vi "Trainging_Program_redesign_TV_White.vi"() -> ()   [LabVIEW 2014]
uses:
  <vilib>/Utility/file.llb/Write To Spreadsheet File (I64).vi
  <vilib>/Utility/file.llb/Write To Spreadsheet File (DBL).vi
  NeuroSky_Dll_Call/Debug/NeuroSky_Dll_Call.dll
panel:
  out "큐사인":bool
  out "실험종료":bool=TRUE
  out "icon_전원":bool
  out "icon_음향업":bool
  out "icon_체널업":bool
  out "icon_음향다운":bool
  out "icon_체널다운":bool=TRUE
  out "icon_전체종료":bool
  out "error out":errorcluster={"status"=TRUE, "code"=10, "source"="Create Folder in Trainging_Set_For_ LDA_Matrix_RSVP.vi<APPEND>\nC:\\Emotion_Research\\_Training_Test(LDA)\\2014-08-30"}
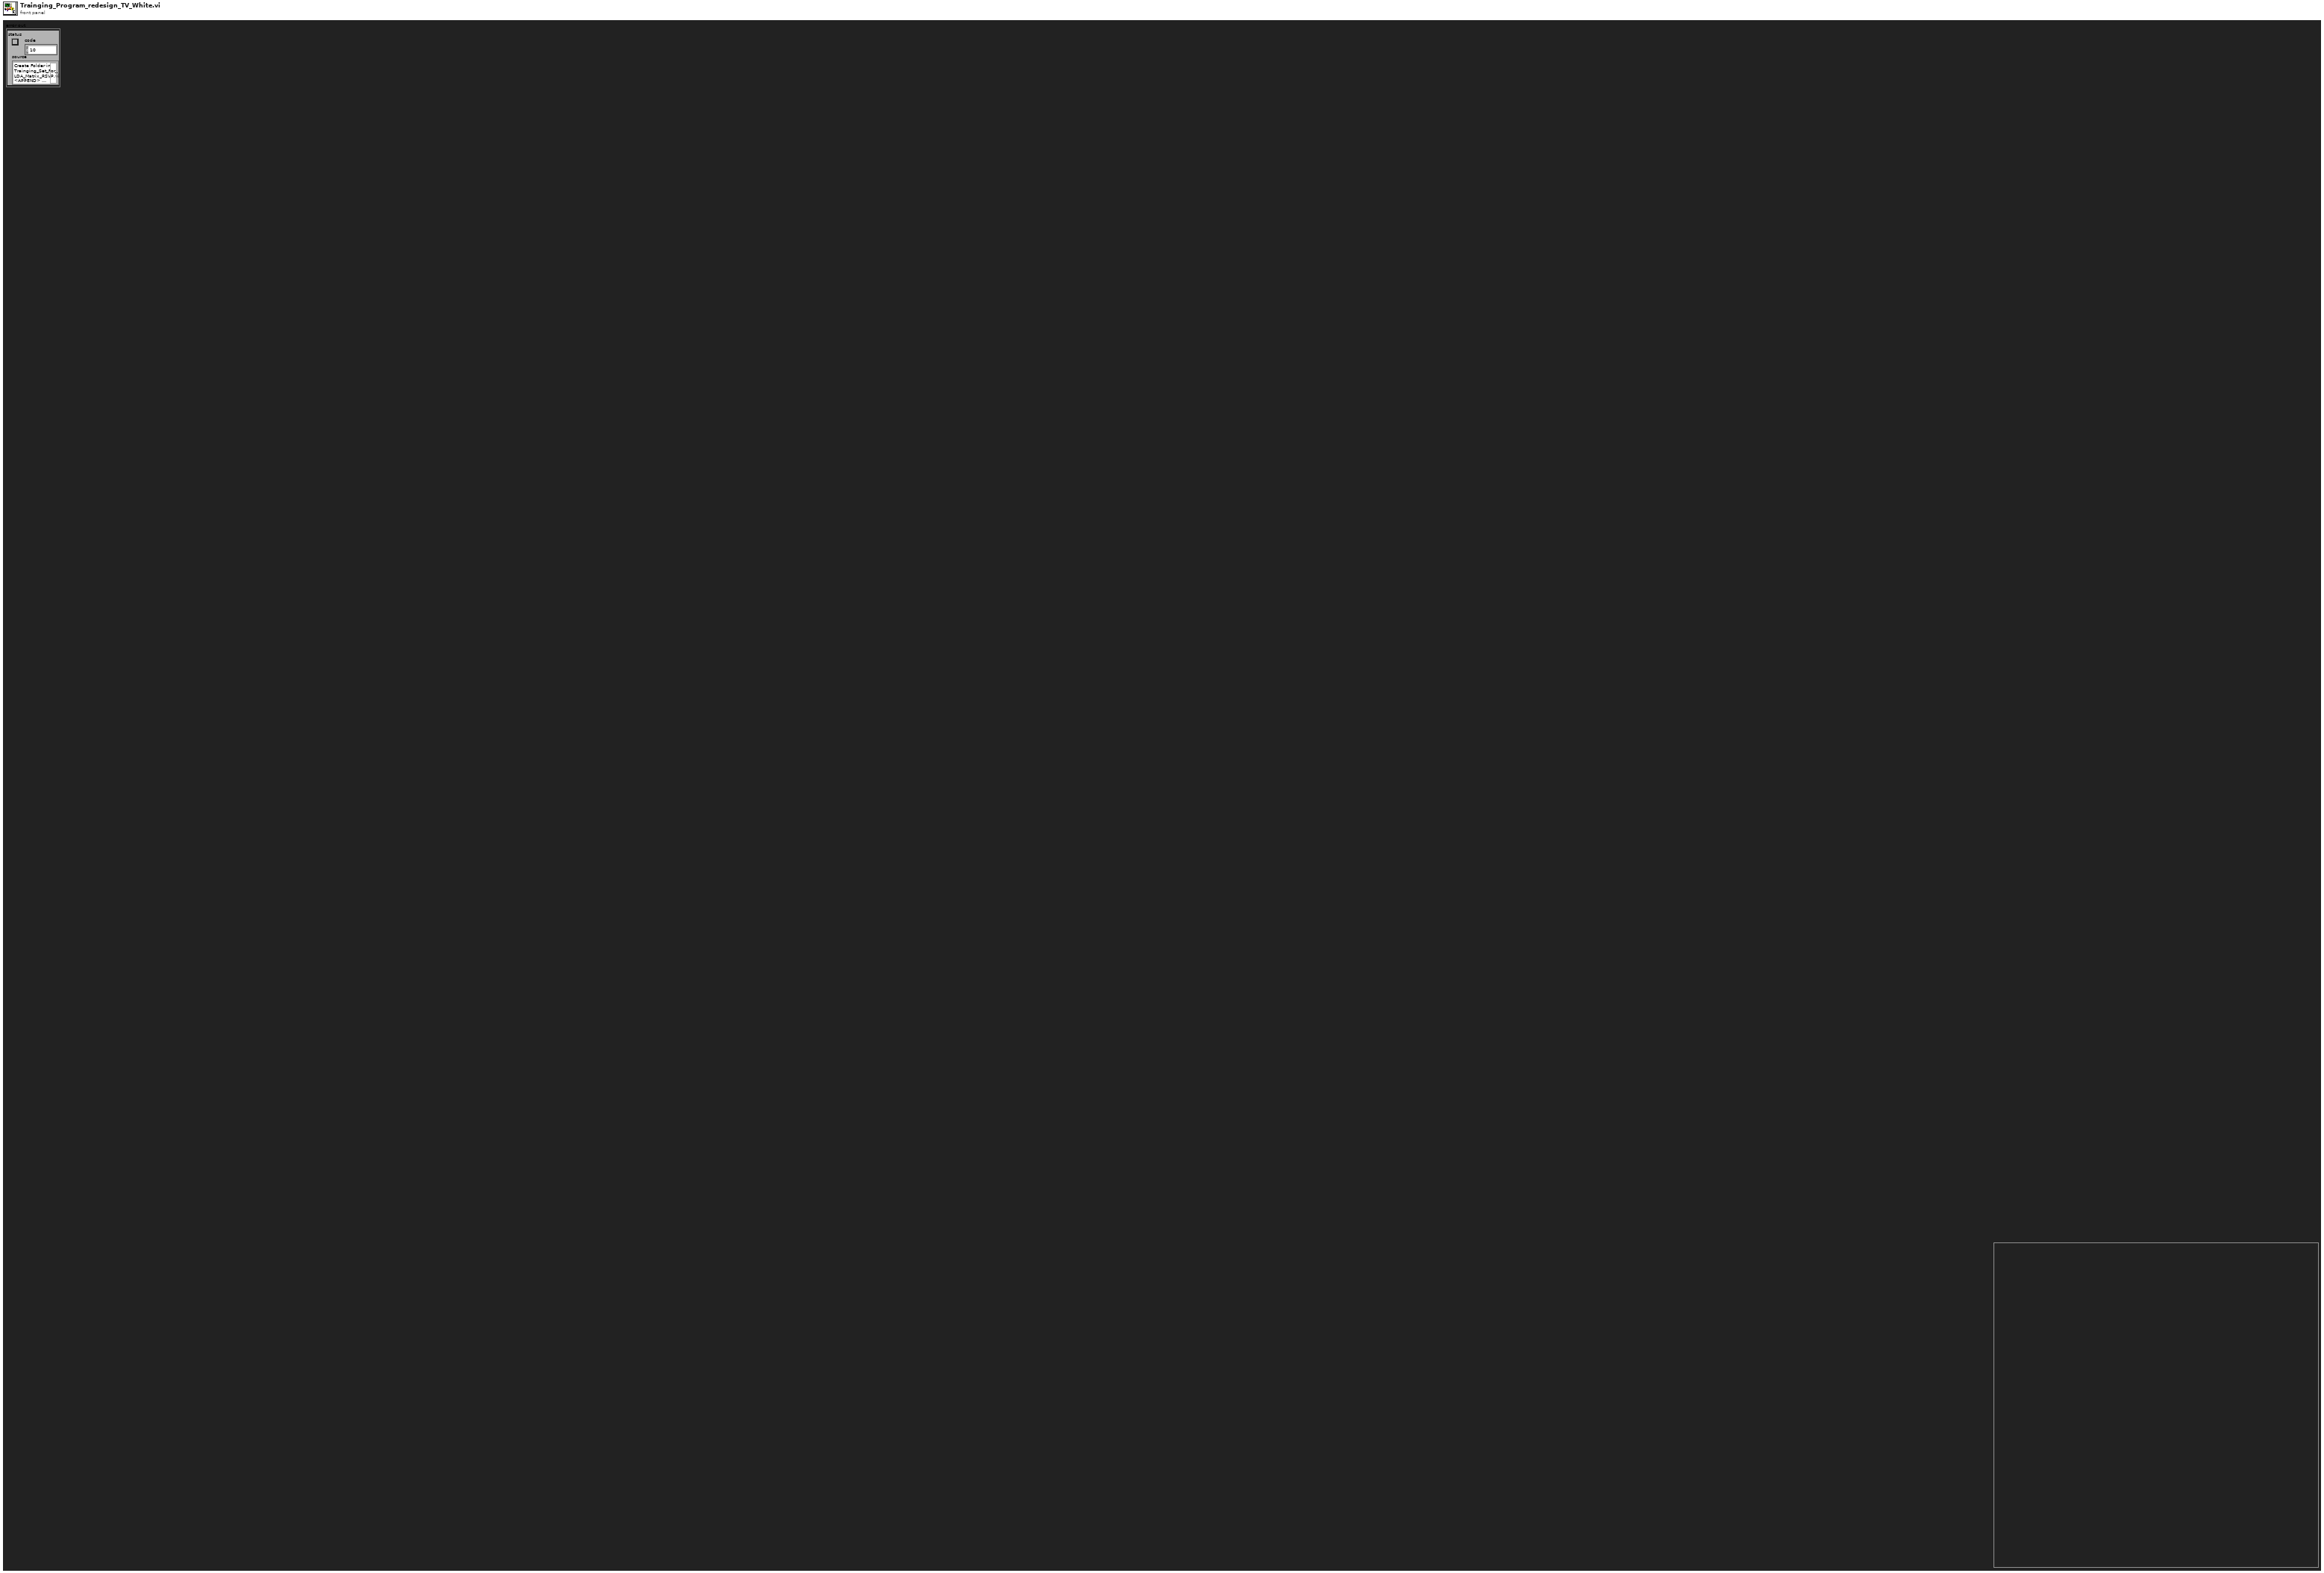
[diagram p1: front panel]
types:
  T1 = typedef "NI_Matrix.lvlib/RealMatrix.ctl" = dbl[][]
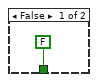
[diagram p2: hidden frame]
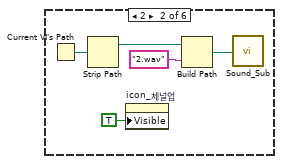
[diagram p3: hidden frame]
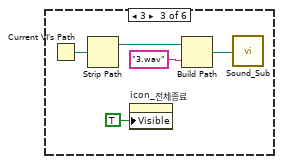
[diagram p4: hidden frame]
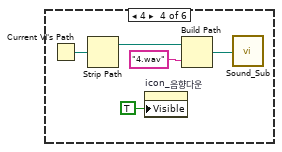
[diagram p5: hidden frame]
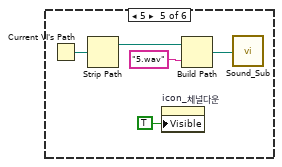
[diagram p6: hidden frame]
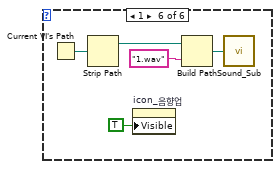
[diagram p7: hidden frame]
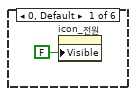
[diagram p8: hidden frame]
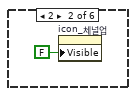
[diagram p9: hidden frame]
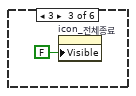
[diagram p10: hidden frame]
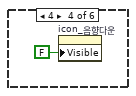
[diagram p11: hidden frame]
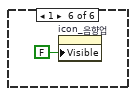
[diagram p12: hidden frame]
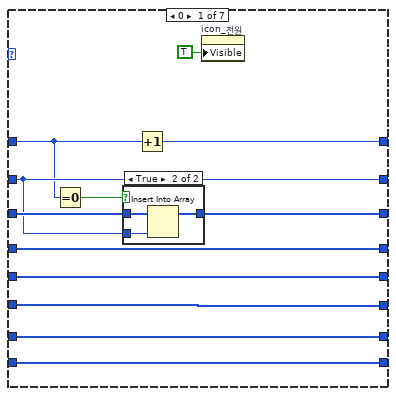
[diagram p14: hidden frame]
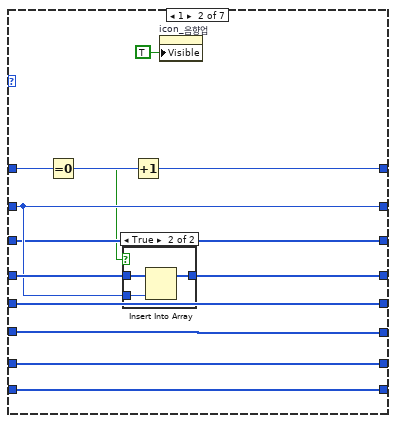
[diagram p16: hidden frame]
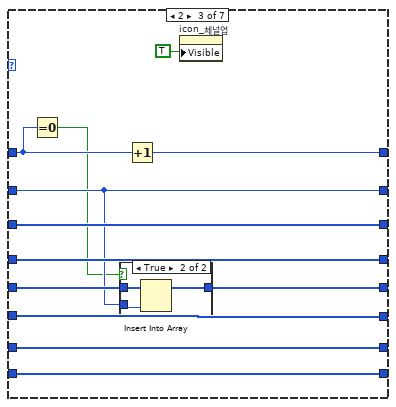
[diagram p18: hidden frame]
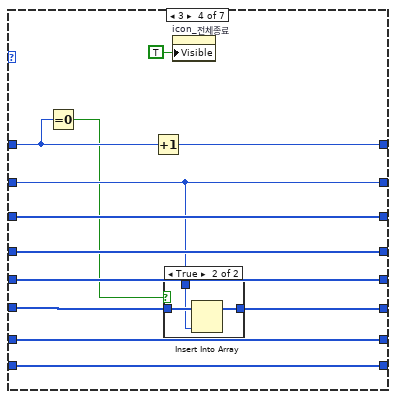
[diagram p20: hidden frame]
diagram:
  w8 = 500 ("Position:Left")
  w1 = FALSE ("Visible")
  # "0 = 온도/전원\n1 = 자판/음향업\n2 = 침대/체널업\n3 = 용변/전체종료\n4 = 기계/음향다운\n5 = 응급/체널다운"
  n1 = property on="icon_음향다운" class="Bool (strict)"("Left"=w8, "Top"=w8) -> ()  [unwired: 2 in, 2 out]
  n2 = property on="icon_음향업" class="Bool (strict)"("Left"=w8, "Top"=w8) -> ()  [unwired: 2 in, 2 out]
  n3 = property on="icon_체널업" class="Bool (strict)"("Left"=w8, "Top"=w8) -> ()  [unwired: 2 in, 2 out]
  n4 = property on="icon_체널다운" class="Bool (strict)"("Left"=w8, "Top"=w8) -> ()  [unwired: 2 in, 2 out]
  n5 = property on="icon_전원" class="Bool (strict)"("Left"=w8, "Top"=w8) -> ()  [unwired: 2 in, 2 out]
  n6 = property on="icon_전체종료" class="Bool (strict)"("Left"=w8, "Top"=w8) -> ()  [unwired: 2 in, 2 out]
  n7 = property on="실험종료" class="Bool (strict)"("Left"=200 ("Position:Left"), "Top"=600 ("Position:Top")) -> ()  [unwired: 2 in, 2 out]
  n8 = property on="큐사인" class="Bool (strict)"("Left"=w8, "Top"=w8) -> ()  [unwired: 2 in, 2 out]
  n9 = property on="큐사인" class="Bool (strict)"("Visible"=w1) -> ()  [unwired: 2 in, 2 out]
  n10 = property on="실험종료" class="Bool (strict)"("Visible"=w1) -> ()  [unwired: 2 in, 2 out]
  n11 = property on="icon_음향다운" class="Bool (strict)"("Visible"=w1) -> ()  [unwired: 2 in, 2 out]
  n12 = property on="icon_전원" class="Bool (strict)"("Visible"=w1) -> ()  [unwired: 2 in, 2 out]
  n13 = property on="icon_음향업" class="Bool (strict)"("Visible"=w1) -> ()  [unwired: 2 in, 2 out]
  n14 = property on="icon_체널업" class="Bool (strict)"("Visible"=w1) -> ()  [unwired: 2 in, 2 out]
  n15 = property on="icon_체널다운" class="Bool (strict)"("Visible"=w1) -> ()  [unwired: 2 in, 2 out]
  n16 = property on="icon_전체종료" class="Bool (strict)"("Visible"=w1) -> ()  [unwired: 2 in, 2 out]
  n17 = flat-sequence {
    tunnel: [w32] -> w31
    tunnel: w31 -> [w46]
    tunnel: [w46] -> w30
    tunnel: [w45] -> w29
    tunnel: w30 -> [w62]
    tunnel: w29 -> [w58]
    tunnel: [w62] -> w28
    tunnel: [w52] -> w27
    tunnel: [w57] -> w26
    tunnel: [w56] -> w25
    tunnel: w28 -> [w371]
    tunnel: w27 -> [w368]
    tunnel: w26 -> [w369]
    tunnel: w25 -> [w370]
    tunnel: [w371] -> w24
    tunnel: [w368] -> w23
    tunnel: [w369] -> w22
    tunnel: [w370] -> w21
    tunnel: w24 -> [w389]
    tunnel: w23 -> [w393]
    tunnel: w22 -> [w401]
    tunnel: w21 -> [w400]
    tunnel: [w388] -> w20
    tunnel: [w387] -> w19
    tunnel: [w389] -> w18
    tunnel: [w388] -> w6
    tunnel: [w387] -> w5
    tunnel: w20 -> [w418]
    tunnel: w19 -> [w428]
    tunnel: w18 -> [w413]
    tunnel: [w413] -> w17
    tunnel: w6 -> [w419]
    tunnel: w5 -> [w417]
    tunnel: [w419] -> w4
    tunnel: [w417] -> w3
    tunnel: w17 -> [w440]
    tunnel: w4 -> [w451]
    tunnel: w3 -> [w450]
    frame #0 {
      n18 = Get Date/Time In Seconds() -> (seconds since 1Jan1904=w37:timestamp)
      n19 = global read "Control_Panel_정리.vi" "피험자 이름"() -> (w33:string)
      n20 = Get Date/Time String(seconds (now)=w37) -> (date string=w36:string)  [unwired: 2 in, 1 out]
      n21 = Concatenate Strings("Emotion_Research\\" ("string"), w33, "_Training_Test(LDA)\\" ("문자열")) -> (w41:string)
      n22 = Concatenate Strings(w41, w36) -> (w39:string)
      n23 = Build Path(base path=path "C:/" ("path"), name or relative path=w39) -> (appended path=w38:path)
      n24 = Create Folder(path (use dialog)=w38) -> (created path=w32:path, error out=→"error out":errorcluster)  [unwired: 2 in, 1 out]
    }
    frame #1 {
      n25 = while {
        stop <- w47 stop-if-true
        n26 = global read "Control_Panel_정리.vi" "Start"() -> (w48:bool)
        n27 = case shown="True" w48 {
          tunnel: [FALSE ("Connected") w50] -> w47
          frame False {
          }
          frame True {
            n28 = call "Control_module.vi"("Turn on"=TRUE ("Device Control Enabled")) -> ("Connected"=w50:bool)
            n29 = global write "Control_Panel_정리.vi" "Device Control Enabled"(w50) -> ()
          }
        }
      }
      n30 = global read "Control_Panel_정리.vi" "Experimentation_num"() -> (w44:i32)
      n31 = global read "Control_Panel_정리.vi" "Random_num"() -> (w43:i32)
      n32 = call "Random2.vi"("Random_num"=w43, "전체횟수"=w44) -> ("배열"=w45:i32[])
    }
    frame #2 {
      n33 = global write "Control_Panel_정리.vi" "Acquisition Mode"(TRUE ("Device Control Enabled")) -> ()
      n34 = global write "Control_Panel_정리.vi" "Device Control Enabled"(FALSE ("Device Control Enabled")) -> ()
      n35 = while {
        tunnel: w58 -> [w107]
        shift-right: [w102] -> _
        shift-left: 0 ("y") -> [w103]
        shift-right: [w101] -> w56
        shift-left: i32[] [] ("subarray") -> [w89]
        shift-right: [w99] -> w52
        shift-left: dbl[] [] -> [w100]
        shift-right: [w92] -> w57
        shift-left: i32[][] [] -> [w88]
        i -> [w98]
        stop <- w97 stop-if-true
        # "현재타겟에 해당하는 \nflash order 만 가져옴"
        n36 = flat-sequence {
          tunnel: [w111] -> w78
          tunnel: w107 -> [w113]
          tunnel: w98 -> [w112]
          tunnel: [w114] -> w76
          tunnel: w103 -> [w114]
          tunnel: [w108] -> w74
          tunnel: w78 -> [w147]
          tunnel: [w147] -> w77
          tunnel: w76 -> [w146]
          tunnel: [w146] -> w75
          tunnel: w74 -> [w145]
          tunnel: [w145] -> w73
          tunnel: w77 -> [w157]
          tunnel: [w157] -> w81
          tunnel: w75 -> [w156]
          tunnel: [w156] -> w80
          tunnel: w73 -> [w155]
          tunnel: [w155] -> w79
          tunnel: w81 -> [w161]
          tunnel: [w161] -> w72
          tunnel: w80 -> [w160]
          tunnel: [w160] -> w70
          tunnel: w79 -> [w159]
          tunnel: [w159] -> w68
          tunnel: w72 -> [w178]
          tunnel: [w178] -> w71
          tunnel: w70 -> [w177]
          tunnel: [w177] -> w69
          tunnel: w68 -> [w176]
          tunnel: [w176] -> w67
          tunnel: w71 -> [w196]
          tunnel: w69 -> [w193]
          tunnel: w67 -> [w187]
          tunnel: [w187] -> w85
          tunnel: [w189] -> w84
          tunnel: [w179] -> w83
          tunnel: [w192] -> w82
          tunnel: w85 -> [w360]
          tunnel: w84 -> [w359]
          tunnel: w83 -> [w358]
          tunnel: w82 -> [w357]
          tunnel: [w360] -> w66
          tunnel: [w359] -> w65
          tunnel: [w358] -> w64
          tunnel: [w357] -> w63
          tunnel: [w364] -> w90
          tunnel: [w365] -> w102
          tunnel: [w366] -> w95
          tunnel: [w367] -> w93
          tunnel: w66 -> [w367]
          tunnel: w65 -> [w366]
          tunnel: w64 -> [w365]
          tunnel: w63 -> [w364]
          frame #0 {
            # "타겟 순서"
            # "결과로 만들어지는 배열은 일차원배열로\n출력되면 랜덤 숫자는 0부터 시작함"
            n37 = global read "Control_Panel_정리.vi" "Random_num"() -> (w109:i32)
            n38 = global read "Control_Panel_정리.vi" "Flash_Repeat"() -> (w110:i32)
            n39 = Index Array(array=w113, index=w112) -> (element=w108:i32)
            n40 = case shown="0, Default" w108 {
              frame 0, Default {
                n41 = Current VI's Path() -> (path=w117:path)
                n42 = Strip Path(path=w117) -> (stripped path=w118:path)  [unwired: 1 out]
                n43 = property on="icon_전원" class="Bool (strict)"("Visible"=TRUE) -> ()  [unwired: 2 in, 2 out]
                n44 = Build Path(base path=w118, name or relative path="0.wav" ("이름 또는 상대 경로")) -> (appended path=w116:path)
                n45 = call "Sound_Sub.vi"("path"=w116) -> ()
              }
              frame 2 {
                n46 = Current VI's Path() -> (path=w121:path)
                n47 = Strip Path(path=w121) -> (stripped path=w122:path)  [unwired: 1 out]
                n48 = property on="icon_체널업" class="Bool (strict)"("Visible"=TRUE) -> ()  [unwired: 2 in, 2 out]
                n49 = Build Path(base path=w122, name or relative path="2.wav" ("이름 또는 상대 경로")) -> (appended path=w124:path)
                n50 = call "Sound_Sub.vi"("path"=w124) -> ()
              }
              frame 3 {
                n51 = Current VI's Path() -> (path=w126:path)
                n52 = Strip Path(path=w126) -> (stripped path=w127:path)  [unwired: 1 out]
                n53 = property on="icon_전체종료" class="Bool (strict)"("Visible"=TRUE) -> ()  [unwired: 2 in, 2 out]
                n54 = Build Path(base path=w127, name or relative path="3.wav" ("이름 또는 상대 경로")) -> (appended path=w129:path)
                n55 = call "Sound_Sub.vi"("path"=w129) -> ()
              }
              frame 4 {
                n56 = Current VI's Path() -> (path=w131:path)
                n57 = Strip Path(path=w131) -> (stripped path=w132:path)  [unwired: 1 out]
                n58 = property on="icon_음향다운" class="Bool (strict)"("Visible"=TRUE) -> ()  [unwired: 2 in, 2 out]
                n59 = Build Path(base path=w132, name or relative path="4.wav" ("이름 또는 상대 경로")) -> (appended path=w134:path)
                n60 = call "Sound_Sub.vi"("path"=w134) -> ()
              }
              frame 5 {
                n61 = Current VI's Path() -> (path=w136:path)
                n62 = Strip Path(path=w136) -> (stripped path=w137:path)  [unwired: 1 out]
                n63 = property on="icon_체널다운" class="Bool (strict)"("Visible"=TRUE) -> ()  [unwired: 2 in, 2 out]
                n64 = Build Path(base path=w137, name or relative path="5.wav" ("이름 또는 상대 경로")) -> (appended path=w139:path)
                n65 = call "Sound_Sub.vi"("path"=w139) -> ()
              }
              frame 1 {
                n66 = Current VI's Path() -> (path=w142:path)
                n67 = Strip Path(path=w142) -> (stripped path=w143:path)  [unwired: 1 out]
                n68 = property on="icon_음향업" class="Bool (strict)"("Visible"=TRUE) -> ()  [unwired: 2 in, 2 out]
                n69 = Build Path(base path=w143, name or relative path="1.wav" ("이름 또는 상대 경로")) -> (appended path=w141:path)
                n70 = call "Sound_Sub.vi"("path"=w141) -> ()
              }
            }
            n71 = call "Random2.vi"("Random_num"=w109, "전체횟수"=w110) -> ("배열"=w111:i32[])
          }
          frame #1 {
            n72 = case shown="5" w145 {
              frame 0, Default {
                n73 = property on="icon_전원" class="Bool (strict)"("Visible"=FALSE) -> ()  [unwired: 2 in, 2 out]
              }
              frame 2 {
                n74 = property on="icon_체널업" class="Bool (strict)"("Visible"=FALSE) -> ()  [unwired: 2 in, 2 out]
              }
              frame 3 {
                n75 = property on="icon_전체종료" class="Bool (strict)"("Visible"=FALSE) -> ()  [unwired: 2 in, 2 out]
              }
              frame 4 {
                n76 = property on="icon_음향다운" class="Bool (strict)"("Visible"=FALSE) -> ()  [unwired: 2 in, 2 out]
              }
              frame 5 {
                n77 = property on="icon_체널다운" class="Bool (strict)"("Visible"=FALSE) -> ()  [unwired: 2 in, 2 out]
              }
              frame 1 {
                n78 = property on="icon_음향업" class="Bool (strict)"("Visible"=FALSE) -> ()  [unwired: 2 in, 2 out]
              }
            }
          }
          frame #2 {
            n79 = property on="큐사인" class="Bool (strict)"("Visible"=TRUE) -> ()  [unwired: 2 in, 2 out]
          }
          frame #3 {
            # "1. NeuroSky의 경우 전송되지 않은 데이터도 축적하여 FIFO 방식으로 GetValue() 함수를 호출할때 한개의 값씩 보내는 방식을 취한다. 현재 MindWave Mobile은 Sampling rate가 512 Hz이며, 2ms의 wait 를 주어 값을 받을 경우 초당 12 sample씩 데이터가 밀리게 된다 \n\n                512 sample/sec - 500 sample /sec = 12 sample /sec\n\n따라서 wait를 주어 500 sample로 맞추는 방식보다 GetValue를 data 값이 정상으로 나올때까지 while로 지속적으로 호출하는 방식으로 syncrhonize 하는 것이 좋다.\n\n2. NeuroSky가 데이터를 전송하지 않더라고 수집을 하기 때문에 Connect()를 통해 통신이 연결된 후 GetValue()를 통해 값을 호출 할때 GetValue()사이에 시간 간격이 생기면 값이 밀리게 된다. 따라서 값을 호출하지 않는 경우 Disconnect()를 통해 통신을 끊어야 Synchornize를 할 수 있다.\n\n3. 통신을 다시 할 경우 1051개의 쓰레기 데이터를 전송하기 때문에 이 값은 dump해버리도록 한다."
            n80 = global read "Control_Panel_정리.vi" "Connected"() -> (w158:bool)
            n81 = case shown="False" w158 {
              frame False {
                n82 = flat-sequence {
                  frame #0 {
                    n83 = dll-call lib="PTH2uabs CUsersJaehongDesktop연구_programNeuroSky_최종본NeuroSky_Dll_CallDebugNeuroSky_Dll_Call.dll" fn="Connect"() -> ()  [unwired: 4 in, 2 out]
                  }
                  frame #1 {
                    n84 = global write "Control_Panel_정리.vi" "Connection"("Reconnected") -> ()
                    n85 = global write "Control_Panel_정리.vi" "Connected"(TRUE ("Connected")) -> ()
                  }
                  frame #2 {
                    n86 = for {
                      N: 1200 -> [_]
                      tunnel: [w166] -> w164 mode=indexing
                      n87 = while {
                        tunnel: [w168] -> w166
                        stop <- w167 stop-if-true
                        n88 = Initialize Array(0.0 ("element"), 100 ("dimension size")) -> (w173:dbl[])
                        n89 = dll-call lib="PTH2uabs CUsersJaehongDesktop연구_programNeuroSky_최종본NeuroSky_Dll_CallDebugNeuroSky_Dll_Call.dll" fn="GetValue"("result"=w173) -> ("result"=w174:dbl[])  [unwired: 4 in, 2 out]
                        n90 = Index Array(array=w174, index=1) -> (element=w168:dbl)
                        n91 = Greater?(x=w168, y=-100000.0) -> (0:w167:bool)
                      }
                    }
                    n92 = global write "Control_Panel_정리.vi" "Dump"(w164) -> ()
                  }
                }
              }
              frame True {
              }
            }
          }
          frame #4 {
            n93 = property on="큐사인" class="Bool (strict)"("Visible"=FALSE) -> ()  [unwired: 2 in, 2 out]
          }
          frame #5 {
            w188 = i32[] []
            # "random_repeat * random_num"
            # "마지막 자극제시 후\n1초데이터를 받기 위한 부분\n(960ms)"
            n94 = while {
              tunnel: w196 -> [w234]
              shift-right: [w197] -> w192
              shift-left: dbl[] [] -> [w199]
              shift-right: [w233] -> w181
              shift-left: w188 -> [w232]
              shift-right: [w230] -> w182
              shift-left: w188 -> [w231]
              shift-right: [w228] -> w183
              shift-left: w188 -> [w229]
              shift-right: [w226] -> w184
              shift-left: w188 -> [w227]
              shift-right: [w224] -> w185
              shift-left: w188 -> [w225]
              shift-right: [w223] -> w186
              shift-left: w188 -> [w215]
              shift-right: [w221] -> w179
              shift-left: w193 -> [w222]
              shift-right: [w220] -> _
              shift-left: 0 -> [w218]
              shift-right: [w216] -> _
              shift-left: 0 ("y") -> [w217]
              tunnel: 8 -> [w198]
              i -> [w219]
              stop <- w200 stop-if-true
              # "ITR =  ~240ms"
              # "0 = 온도\n1 = 자판\n2 = 침대\n3 = 용변 \n4 = 기계 \n5 = 응급"
              n95 = flat-sequence {
                tunnel: [w345] -> w197
                tunnel: w199 -> [w343]
                frame #0 {
                  # "Packet 단위로 송신\n이는 반짝이는 효과를 주기 위함\n1 Packet = 20 data (~40ms)"
                  n96 = for {
                    N: 20 -> [_]
                    tunnel: [w346] -> w344 mode=indexing
                    n97 = while {
                      tunnel: [w348] -> w346
                      stop <- w347 stop-if-true
                      n98 = Initialize Array(0.0 ("element"), 100 ("dimension size")) -> (w354:dbl[])
                      n99 = dll-call lib="PTH2uabs CUsersJaehongDesktop연구_programNeuroSky_최종본NeuroSky_Dll_CallDebugNeuroSky_Dll_Call.dll" fn="GetValue"("result"=w354) -> ("errCode"=w350:string, "result"=w355:dbl[])  [unwired: 3 in, 2 out]
                      n100 = global write "Control_Panel_정리.vi" "Value Achieving Status"(w350) -> ()
                      n101 = Index Array(array=w355, index=1) -> (element=w348:dbl)
                      n102 = Greater?(x=w348, y=-100000.0) -> (0:w347:bool)
                    }
                    n103 = global write "Control_Panel_정리.vi" "웨이브폼 차트"(w346) -> ()
                  }
                  n104 = Build Array (concatenate)(w343, w344) -> (w345:dbl[])
                }
              }
              n105 = global read "Control_Panel_정리.vi" "Random_num"() -> (w202:i32)
              n106 = global read "Control_Panel_정리.vi" "Flash_Repeat"() -> (w203:i32)
              n107 = Increment(x=w219) -> (x+1=w205:i32)
              n108 = Quotient & Remainder(x=w205, y=6) -> (x-y*floor(x/y)=w210:i32)  [unwired: 1 out]
              n109 = Equal To 0?(x=w210) -> (x = 0?=w208:bool)
              n110 = Multiply(x=w203, y=w202) -> (x*y=w201:i32)
              n111 = Add(x=w198, y=w201) -> (x+y=w214:i32)
              n112 = Greater Or Equal?(x=w218, y=w201) -> (x >= y?=w207:bool)
              n113 = Increment(x=w218) -> (x+1=w209:i32)
              n114 = Increment(x=w222) -> (x+1=w212:i32)
              n115 = Equal?(x=w218, y=w214) -> (x = y?=w200:bool)
              n116 = Index Array(array=w234, index=w218) -> (element=w204:i32)
              n117 = Or(x=w208, y=w207) -> (x .or. y?=w206:bool)
              n118 = Select(t=w209, s=w208, f=w218) -> (s? t:f=w220:i32)
              n119 = Select(t=w202, s=w206, f=w204) -> (s? t:f=w213:i32)
              n120 = case shown="6, Default" w213 {
                tunnel: w212 -> [w240 w256 w271 w287 w303 w320 w335]
                tunnel: [w245 w253 w278 w294 w310 w326 w341] -> w233
                tunnel: w232 -> [w246 w253 w278 w294 w310 w326 w341]
                tunnel: w231 -> [w244 w262 w275 w291 w307 w324 w340]
                tunnel: [w244 w261 w275 w291 w307 w324 w340] -> w230
                tunnel: w229 -> [w243 w260 w277 w290 w306 w323 w339]
                tunnel: [w243 w260 w276 w290 w306 w323 w339] -> w228
                tunnel: w227 -> [w242 w259 w274 w293 w305 w322 w338]
                tunnel: [w242 w259 w274 w292 w305 w322 w338] -> w226
                tunnel: w225 -> [w241 w258 w273 w289 w309 w321 w337]
                tunnel: [w241 w258 w273 w289 w308 w321 w337] -> w224
                tunnel: w215 -> [w237 w257 w272 w288 w304 w325 w336]
                tunnel: [w237 w257 w272 w288 w304 w317 w336] -> w223
                tunnel: [w240 w256 w271 w287 w303 w320 w335] -> w221
                tunnel: w217 -> [w239 w255 w270 w285 w302 w318 _]
                tunnel: [w238 w254 w269 w286 w301 w319 0] -> w216
                frame 0 {
                  n121 = Equal To 0?(x=w239) -> (x = 0?=w235:bool)
                  n122 = case shown="True" w235 {
                    tunnel: w246 -> [w247 w250]
                    tunnel: [w247 w249] -> w245
                    tunnel: w240 -> [_ w248]
                    frame False {
                    }
                    frame True {
                      n123 = Insert Into Array(array=w250, new element=w248) -> (w249:i32[])  [unwired: 1 in]
                    }
                  }
                  n124 = Increment(x=w239) -> (x+1=w238:i32)
                  n125 = property on="icon_전원" class="Bool (strict)"("Visible"=TRUE) -> ()  [unwired: 2 in, 2 out]
                }
                frame 1 {
                  n126 = Equal To 0?(x=w255) -> (x = 0?=w251:bool)
                  n127 = case shown="True" w251 {
                    tunnel: w262 -> [w263 w266]
                    tunnel: [w263 w265] -> w261
                    tunnel: w256 -> [_ w264]
                    frame False {
                    }
                    frame True {
                      n128 = Insert Into Array(array=w266, new element=w264) -> (w265:i32[])  [unwired: 1 in]
                    }
                  }
                  n129 = Increment(x=w255) -> (x+1=w254:i32)
                  n130 = property on="icon_음향업" class="Bool (strict)"("Visible"=TRUE) -> ()  [unwired: 2 in, 2 out]
                }
                frame 2 {
                  n131 = Equal To 0?(x=w270) -> (x = 0?=w267:bool)
                  n132 = case shown="True" w267 {
                    tunnel: w277 -> [w279 w282]
                    tunnel: [w279 w281] -> w276
                    tunnel: w271 -> [_ w280]
                    frame False {
                    }
                    frame True {
                      n133 = Insert Into Array(array=w282, new element=w280) -> (w281:i32[])  [unwired: 1 in]
                    }
                  }
                  n134 = Increment(x=w270) -> (x+1=w269:i32)
                  n135 = property on="icon_체널업" class="Bool (strict)"("Visible"=TRUE) -> ()  [unwired: 2 in, 2 out]
                }
                frame 3 {
                  n136 = Equal To 0?(x=w285) -> (x = 0?=w283:bool)
                  n137 = Increment(x=w285) -> (x+1=w286:i32)
                  n138 = case shown="True" w283 {
                    tunnel: w293 -> [w295 w298]
                    tunnel: [w295 w297] -> w292
                    tunnel: w287 -> [_ w296]
                    frame False {
                    }
                    frame True {
                      n139 = Insert Into Array(array=w298, new element=w296) -> (w297:i32[])  [unwired: 1 in]
                    }
                  }
                  n140 = property on="icon_전체종료" class="Bool (strict)"("Visible"=TRUE) -> ()  [unwired: 2 in, 2 out]
                }
                frame 4 {
                  n141 = Equal To 0?(x=w302) -> (x = 0?=w299:bool)
                  n142 = case shown="False" w299 {
                    tunnel: w309 -> [w311 w314]
                    tunnel: [w311 w313] -> w308
                    tunnel: w303 -> [_ w312]
                    frame False {
                    }
                    frame True {
                      n143 = Insert Into Array(array=w314, new element=w312) -> (w313:i32[])  [unwired: 1 in]
                    }
                  }
                  n144 = Increment(x=w302) -> (x+1=w301:i32)
                  n145 = property on="icon_음향다운" class="Bool (strict)"("Visible"=TRUE) -> ()  [unwired: 2 in, 2 out]
                }
                frame 5 {
                  n146 = Equal To 0?(x=w318) -> (x = 0?=w315:bool)
                  n147 = Increment(x=w318) -> (x+1=w319:i32)
                  n148 = property on="icon_체널다운" class="Bool (strict)"("Visible"=TRUE) -> ()  [unwired: 2 in, 2 out]
                  n149 = case shown="True" w315 {
                    tunnel: w325 -> [w327 w330]
                    tunnel: [w327 w329] -> w317
                    tunnel: w320 -> [_ w328]
                    frame False {
                    }
                    frame True {
                      n150 = Insert Into Array(array=w330, new element=w328) -> (w329:i32[])  [unwired: 1 in]
                    }
                  }
                }
                frame 6, Default {
                  w332 = FALSE ("Visible")
                  w331 = FALSE ("Visible")
                  w333 = FALSE ("Visible")
                  n151 = property on="icon_체널다운" class="Bool (strict)"("Visible"=w333) -> ()  [unwired: 2 in, 2 out]
                  n152 = property on="icon_전체종료" class="Bool (strict)"("Visible"=w333) -> ()  [unwired: 2 in, 2 out]
                  n153 = property on="icon_음향다운" class="Bool (strict)"("Visible"=w331) -> ()  [unwired: 2 in, 2 out]
                  n154 = property on="icon_전원" class="Bool (strict)"("Visible"=w331) -> ()  [unwired: 2 in, 2 out]
                  n155 = property on="icon_체널업" class="Bool (strict)"("Visible"=w332) -> ()  [unwired: 2 in, 2 out]
                  n156 = property on="icon_음향업" class="Bool (strict)"("Visible"=w332) -> ()  [unwired: 2 in, 2 out]
                }
              }
            }
            n157 = Build Array(w181, w182, w183, w184, w185, w186) -> (w194:i32[][])
            n158 = Transpose 2D Array(2D array=w194) -> (transposed array=w189:i32[][])
          }
          frame #6 {
            # "1 Iteration이 끝나고 Disconnect하도록 한다. Synchronize를 위한 방법론"
            n159 = global read "Control_Panel_정리.vi" "Connected"() -> (w356:bool)
            n160 = case shown="True" w356 {
              frame False {
              }
              frame True {
                n161 = flat-sequence {
                  frame #0 {
                    n162 = dll-call lib="PTH2uabs CUsersJaehongDesktop연구_programNeuroSky_최종본NeuroSky_Dll_CallDebugNeuroSky_Dll_Call.dll" fn="Disconnect"() -> ()  [unwired: 4 in, 2 out]
                  }
                  frame #1 {
                    n163 = global write "Control_Panel_정리.vi" "Connection"("Disconnected") -> ()
                    n164 = global write "Control_Panel_정리.vi" "Connected"(FALSE ("Connected")) -> ()
                  }
                }
              }
            }
          }
          frame #7 {
            w363 = FALSE ("Visible")
            n165 = property on="icon_음향업" class="Bool (strict)"("Visible"=w363) -> ()  [unwired: 2 in, 2 out]
            n166 = property on="icon_음향다운" class="Bool (strict)"("Visible"=w363) -> ()  [unwired: 2 in, 2 out]
            n167 = property on="icon_체널업" class="Bool (strict)"("Visible"=w363) -> ()  [unwired: 2 in, 2 out]
            n168 = property on="icon_체널다운" class="Bool (strict)"("Visible"=w363) -> ()  [unwired: 2 in, 2 out]
            n169 = property on="icon_전원" class="Bool (strict)"("Visible"=w363) -> ()  [unwired: 2 in, 2 out]
            n170 = property on="icon_전체종료" class="Bool (strict)"("Visible"=w363) -> ()  [unwired: 2 in, 2 out]
          }
        }
        n171 = global read "Control_Panel_정리.vi" "Experimentation_num"() -> (w87:i32)
        n172 = global read "Control_Panel_정리.vi" "Random_num"() -> (w86:i32)
        n173 = Multiply(x=w87, y=w86) -> (x*y=w105:i32)
        n174 = Subtract(x=w105, y=2) -> (x-y=w106:i32)
        n175 = Greater?(x=w98, y=w106) -> (0:w97:bool)
        n176 = Index Array(array=w95, index (col)=w93) -> (element=w96:i32[])  [unwired: 1 in]
        n177 = Insert Into Array(array=w100, new element=w90) -> (w99:dbl[])  [unwired: 1 in]
        n178 = Delete From Array(array=w95, length=1 ("길이"), index (col)=w93) -> (array with subset deleted=w94:i32[][])  [unwired: 1 in, 1 out]
        n179 = Build Array (concatenate)(w88, w94) -> (w92:i32[][])
        n180 = Insert Into Array(array=w89, new element=w96) -> (w101:i32[])  [unwired: 1 in]
      }
    }
    frame #3 {
      # "현재타겟에 해당하는 \nflash order 만 가져옴"
      # "target=stimulus 때의 order만 가져옴"
      n181 = flat-sequence {
        frame #0 {
          n182 = dll-call lib="PTH2uabs CUsersJaehongDesktop연구_programNeuroSky_최종본NeuroSky_Dll_CallDebugNeuroSky_Dll_Call.dll" fn="FreeConnection"() -> ()  [unwired: 4 in, 2 out]
        }
        frame #1 {
          n183 = property on="실험종료" class="Bool (strict)"("Visible"=TRUE) -> ()  [unwired: 2 in, 2 out]
        }
        frame #2 {
          n184 = global write "Control_Panel_정리.vi" "Value Achieving Status"("All Connection terminated,\nExperiment over" ("name or relative path")) -> ()
          n185 = global write "Control_Panel_정리.vi" "Acquisition Mode"(FALSE ("Device Control Enabled")) -> ()
        }
      }
      n186 = Build Path(base path=w371, name or relative path="Brain.txt") -> (appended path=w374:path)
      n187 = Build Path(base path=w371, name or relative path="Target_order.txt") -> (appended path=w377:path)
      n188 = call-poly <vilib>:"Write To Spreadsheet File.vi"("transpose? (no:F)"=TRUE, "1D data"=w370, "file path (dialog if empty)"=w377) -> ()  [unwired: 5 in, 1 out]
      n189 = Build Path(base path=w371, name or relative path="Nontarget_order.txt") -> (appended path=w378:path)
      n190 = call-poly <vilib>:"Write To Spreadsheet File.vi"("format (%.3f)"="%.6f", "1D data"=w368, "file path (dialog if empty)"=w374) -> ()  [unwired: 5 in, 1 out]
      n191 = call-poly <vilib>:"Write To Spreadsheet File.vi"("transpose? (no:F)"=FALSE, "2D data"=w369, "file path (dialog if empty)"=w378) -> ()  [unwired: 5 in, 1 out]
    }
    frame #4 {
      n192 = global read "Control_Panel_정리.vi" "Experimentation_num"() -> (w404:i32)
      n193 = global read "Control_Panel_정리.vi" "Flash_Repeat"() -> (w406:i32)
      n194 = global read "Control_Panel_정리.vi" "Random_num"() -> (w405:i32)
      n195 = global write "Control_Panel_정리.vi" "Communication Stopped"(TRUE ("Device Control Enabled")) -> ()
      n196 = global read "Control_Panel_정리.vi" "Frame Length"() -> (w402:i32)
      n197 = global read "Control_Panel_정리.vi" "rate"() -> (w403:dbl)
      n198 = call "Subvi_Training_Baseline_w_range_w_weight.vi"("Nontarget_Flash_Order"=w401, "Target_Flash_Order"=w400, "samples per channel"=w402, "Brain_data_source"=w393, "rate"=w403, "Experimentation_num"=w404, "Random_num"=w405, "Random_Repeat"=w406) -> ("Target_ERP"=w384:dbl[], "NonTarget"=w387:dbl[][], "Nontarget_ERP"=w385:dbl[], "Target"=w388:dbl[][])
      n199 = Build Path(base path=w389, name or relative path="Nontarget_ERP_AVG.txt") -> (appended path=w391:path)
      n200 = Build Path(base path=w389, name or relative path="Target_ERP_AVG.txt") -> (appended path=w408:path)
      n201 = Build Path(base path=w389, name or relative path="ERP_Parameters_of_Target_prior.txt") -> (appended path=w398:path)
      n202 = Build Path(base path=w389, name or relative path="ERP_Parameters_of_NonTarget_prior.txt") -> (appended path=w395:path)
      n203 = call-poly <vilib>:"Write To Spreadsheet File.vi"("format (%.3f)"="%.6f", "1D data"=w385, "file path (dialog if empty)"=w391) -> ()  [unwired: 5 in, 1 out]
      n204 = call-poly <vilib>:"Write To Spreadsheet File.vi"("format (%.3f)"="%.6f", "1D data"=w384, "file path (dialog if empty)"=w408) -> ()  [unwired: 5 in, 1 out]
      n205 = call-poly <vilib>:"Write To Spreadsheet File.vi"("format (%.3f)"="%.6f", "2D data"=w388, "file path (dialog if empty)"=w398) -> ()  [unwired: 5 in, 1 out]
      n206 = call-poly <vilib>:"Write To Spreadsheet File.vi"("format (%.3f)"="%.6f", "2D data"=w387, "file path (dialog if empty)"=w395) -> ()  [unwired: 5 in, 1 out]
    }
    frame #5 {
      n207 = Array Size(array=w418) -> (size(s)=w431:i32[])
      n208 = Array Size(array=w428) -> (size(s)=w432:i32[])
      n209 = Index Array(array=w431) -> (element=w433:i32)  [unwired: 1 in]
      n210 = Index Array(array=w432) -> (element=w434:i32)  [unwired: 1 in]
      n211 = for {
        N: w434 -> [_]
        tunnel: [1] -> w436 mode=indexing
      }
      n212 = for {
        N: w433 -> [_]
        tunnel: [0] -> w435 mode=indexing
      }
      n213 = Build Array (concatenate)(w435, w436) -> (w427:i32[])
      n214 = Build Array (concatenate)(w418, w428) -> (w429:dbl[][])
      n215 = global read "Control_Panel_정리.vi" "EEG_Channel_Num"() -> (w410:i32)
      n216 = Insert Into Array(array=w429, index (col)=0 ("비활성화된 인덱스 (열)"), new element=w427) -> (w423:dbl[][])  [unwired: 1 in]
      n217 = call "Subvi_Training_LDA.vi"("Input_Data"=w423) -> ("A * B 2"=w421:T1, "A * B"=w422:T1)
      n218 = Initialize Array(0.090909 ("element"), w410) -> (w412:dbl[])
      n219 = Build Array (concatenate)(w422, w421) -> (w420:T1)
      n220 = Build Path(base path=w413, name or relative path="Weight_Vector_prior.txt") -> (appended path=w416:path)
      n221 = Build Path(base path=w413, name or relative path="LDA_Matrix_Value_prior.txt") -> (appended path=w425:path)
      n222 = call-poly <vilib>:"Write To Spreadsheet File.vi"("format (%.3f)"="%.6f", "1D data"=w412, "file path (dialog if empty)"=w416) -> ()  [unwired: 5 in, 1 out]
      n223 = call-poly <vilib>:"Write To Spreadsheet File.vi"("format (%.3f)"="%.6f", "2D data"=w420, "file path (dialog if empty)"=w425) -> ()  [unwired: 5 in, 1 out]
    }
    frame #6 {
      (unwired) "%.6f" ("format (%.3f)")
      # "addpath('C:\\Users\\Jaehong\\Desktop\\연구_program\\libsvm-3.18\\matlab');"
      n224 = call "SWLDA_통합버전용.vi"("premove"=0.05, "penter"=0.01, "ERP_Nontarget"=w450, "ERP_Target"=w451) -> ("in"=w439:dbl[], "LDA_matrix"=w455:T1)  [unwired: 5 in, 1 out]
      n225 = global read "Control_Panel_정리.vi" "EEG_Channel_Num"() -> (w444:i32)
      n226 = global read "Control_Panel_정리.vi" "EEG_Channel_Num"() -> (w454:i32)
      n227 = global read "Control_Panel_정리.vi" "Random_num"() -> (w453:i32)
      n228 = global read "Control_Panel_정리.vi" "Experimentation_num"() -> (w452:i32)
      n229 = Initialize Array(0.090909 ("element"), w444) -> (w446:dbl[])
      n230 = script code="%addpath to the libsvm toolbox\n\naddpath('C:\\Users\\Server\\Desktop\\NeuroSky\\RSVP_NeuroSky\\libsvm-3.18\\matlab');\n\n%read data set(training)\n\nrow_num = chan_num*4;\ncol_num = icon_num*exp_num;\n\nWeight = Weight';\nnonzeros = find(Weight, row_num);\ntarget = reshape(target', row_num, col_num);\ntarget = target.*Weight(:,ones(1,col_num));\ntarget = target(nonzeros,:);\nnontarget = reshape(nontarget', row_num, col_num);\nnontarget = nontarget.*Weight(:,ones(1,col_num));\nnontarget = nontarget(nonzeros,:);\nEEG_train = [target';nontarget']';\nlength = size(target,2);\ntrainLabel = [ones(length,1);-ones(length, 1)];\n\n% Train the SVM\n\nmodel = ...\nsvmtrain(trainLabel, [(1:col_num*2)' EEG_train'*EEG_train], '-c 1 -g 0.07 -b 1 -t 4 -q');\n\n%save model file\nsvm_savemodel(model,'C:\\WORK\\svm_model.model');" ("Script Node")("Weight"=w439, "target"=w450, "nontarget"=w451, "icon_num"=w453, "chan_num"=w454, "exp_num"=w452) -> ()  [unwired: 1 in, 1 out]
      n231 = Build Path(base path=w440, name or relative path="LDA_Matrix_Value_SWLDA.txt") -> (appended path=w458:path)
      n232 = Build Path(base path=w440, name or relative path="in_SWLDA.txt") -> (appended path=w443:path)
      n233 = Build Path(base path=w440, name or relative path="Weight_Vector_SWLDA.txt") -> (appended path=w449:path)
      n234 = call-poly <vilib>:"Write To Spreadsheet File.vi"("2D data"=w455, "file path (dialog if empty)"=w458) -> ()  [unwired: 6 in, 1 out]
      n235 = call-poly <vilib>:"Write To Spreadsheet File.vi"("format (%.3f)"="%.6f", "1D data"=w439, "file path (dialog if empty)"=w443) -> ()  [unwired: 5 in, 1 out]
      n236 = call-poly <vilib>:"Write To Spreadsheet File.vi"("format (%.3f)"="%.6f", "1D data"=w446, "file path (dialog if empty)"=w449) -> ()  [unwired: 5 in, 1 out]
    }
    frame #7 {
      n237 = global write "Control_Panel_정리.vi" "Communication Stopped"(FALSE ("Device Control Enabled")) -> ()
    }
  }
  "icon_전원" <- FALSE ("icon_전원 6")
  "icon_전체종료" <- FALSE ("icon_전체종료")
  "icon_음향업" <- FALSE ("icon_음량업 2")
  "icon_체널다운" <- FALSE ("icon_채널다운")
  "icon_음향다운" <- FALSE ("icon_음량다")
  "icon_체널업" <- FALSE ("icon_채널업")
  "실험종료" <- TRUE ("Boolean")
  "큐사인" <- FALSE ("icon_전원 7")
